vi "Configure Series.vi"(8 "error in (no error)":errorcluster, 10 "Enable Series Mode (T: Enable)":bool=TRUE, 11 "VISA resource name":refnum<visa-resource-name>) -> (0 "error out":errorcluster, 3 "VISA resource name out":refnum<visa-resource-name>)   [LabVIEW 2017, in "BK Precision 913XX.lvlib"]
doc: "Enables or disables series mode for channels 1 and 2.\n\n<B>Note: To enable series mode, tracking or parallel mode must first be disabled using Configure Tracking.vi or Configure Parallel.vi respectively. Otherwise, an error will occur.</B>"
uses:
  <instrlib>/BK Precision 913XX/BK Precision 913XX.lvlib
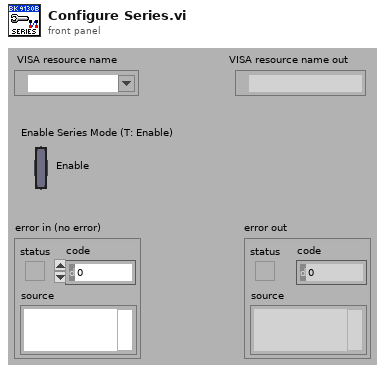
[diagram p1: front panel]
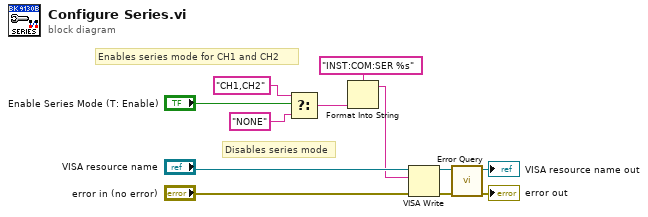
[diagram p0: block diagram]
diagram:
  # "Enables series mode for CH1 and CH2"
  # "Disables series mode"
  n1 = Select(t="CH1,CH2" ("multi-line string"), s="Enable Series Mode (T: Enable)", f="NONE") -> (s? t:f=w5:string)
  n2 = Format Into String(format string="INST:COM:SER %s", w5) -> (resulting string=w2:string)  [unwired: 2 in, 1 out]
  n3 = VISA Write(VISA resource name="VISA resource name", write buffer=w2, error in (no error)="error in (no error)") -> (VISA resource name out=w10:refnum<visa-resource-name>, error out=w9:errorcluster)  [unwired: 1 out]
  n4 = call <instrlib>:"Error Query.vi"("error in (no error)"=w9, "VISA resource name"=w10) -> ("error out"=→"error out":errorcluster, "VISA resource name out"=→"VISA resource name out":refnum<visa-resource-name>)  [unwired: 6 in, 2 out]
